vi "FindMidPointInSelectedJoint.vi"(11 "Joints[]":T2(array[cluster])) -> (0 "output cluster":cluster{"h":i16, "v":i16}, 2 "MidPoint":T1, 3 "Valid?":bool)   [LabVIEW 2014]
uses:
  <vilib>/Utility/miscctls.llb/LVPointTypeDef.ctl
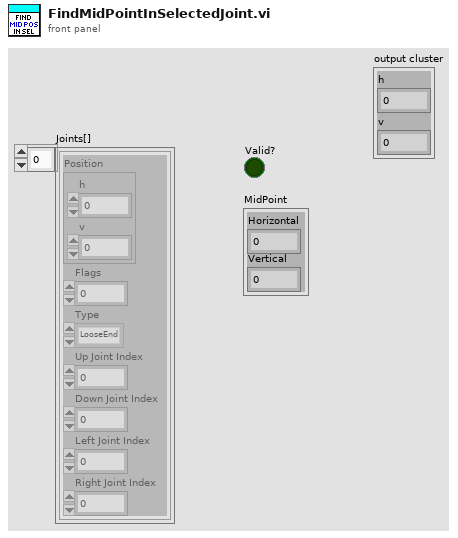
[diagram p1: front panel]
types:
  T1 = typedef "LVPointTypeDef.ctl" = cluster{"Horizontal":i16, "Vertical":i16}
  T2 = cluster{"Position":cluster{"h":i16, "v":i16}, "Flags":i32, "Type":enum32{"LooseEnd", "Endpoint", "Bend", "Junction"}, "Up Joint Index":i16, "Down Joint Index":i16, "Left Joint Index":i16, "Right Joint Index":i16}[]
  T3 = cluster{"Position":cluster{"h":i16, "v":i16}, "Flags":i32, "Type":enum32{"LooseEnd", "Endpoint", "Bend", "Junction"}, "Up Joint Index":i16, "Down Joint Index":i16, "Left Joint Index":i16, "Right Joint Index":i16}
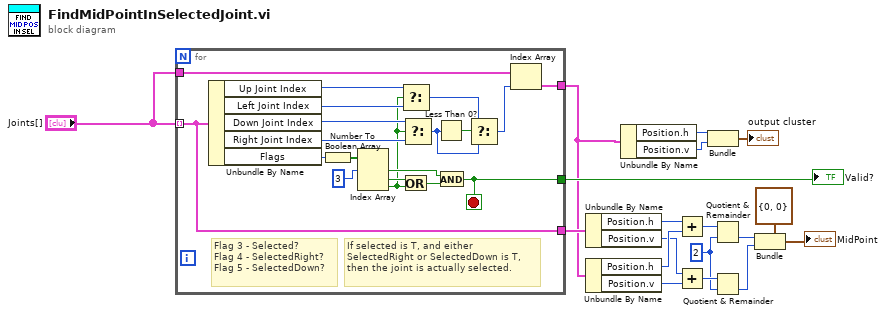
[diagram p0: block diagram]
diagram:
  w10 = i16 2 ("y")
  n1 = for {
    tunnel: "Joints[]" -> [w31] mode=indexing
    tunnel: "Joints[]" -> [w30]
    tunnel: [w31] -> w14
    tunnel: [w29] -> w4
    tunnel: [w19] -> w16
    stop <- w19 stop-if-true
    # "If selected is T, and either SelectedRight or SelectedDown is T, then the joint is actually selected."
    # "Flag 3 - Selected?\nFlag 4 - SelectedRight?\nFlag 5 - SelectedDown?"
    n2 = Unbundle By Name(w31) -> ("Up Joint Index"=w26:i16, "Left Joint Index"=w25:i16, "Down Joint Index"=w28:i16, "Right Joint Index"=w27:i16, "Flags"=w37:i32)
    n3 = Number To Boolean Array(number=w37) -> (Boolean array=w36:bool[])
    n4 = Index Array(array=w36, index #1=3 ("index")) -> (element #1=w32:bool, element #2=w33:bool, element #3=w24:bool)  [unwired: 2 in]
    n5 = Select(t=w26, s=w24, f=w25) -> (s? t:f=w21:i16)
    n6 = Or(x=w33, y=w24) -> (x .or. y?=w34:bool)
    n7 = Select(t=w28, s=w24, f=w27) -> (s? t:f=w20:i16)
    n8 = Less Than 0?(x=w20) -> (x < 0?=w22:bool)
    n9 = And(x=w32, y=w34) -> (x .and. y?=w19:bool)
    n10 = Select(t=w21, s=w22, f=w20) -> (s? t:f=w23:i16)
    n11 = Index Array(array=w30, index=w23) -> (element=w29:T3)
  }
  "Valid?" <- w16
  n12 = Unbundle By Name(w14) -> ("Position.h"=w8:i16, "Position.v"=w6:i16)
  n13 = Unbundle By Name(w4) -> ("Position.h"=w7:i16, "Position.v"=w5:i16)
  n14 = Unbundle By Name(w4) -> ("Position.h"=w3:i16, "Position.v"=w2:i16)
  n15 = Add(x=w8, y=w7) -> (x+y=w13:i16)
  n16 = Add(x=w6, y=w5) -> (x+y=w11:i16)
  n17 = Bundle("h"=w3, "v"=w2) -> (→"output cluster":cluster{"h":i16, "v":i16})  [unwired: 1 in]
  n18 = Quotient & Remainder(x=w13, y=w10) -> (floor(x/y)=w12:i16)  [unwired: 1 out]
  n19 = Quotient & Remainder(x=w11, y=w10) -> (floor(x/y)=w9:i16)  [unwired: 1 out]
  n20 = Bundle(cluster=T1 {"Horizontal"=0, "Vertical"=0} ("Insertion Point"), "Horizontal"=w12, "Vertical"=w9) -> (→"MidPoint":T1)
